vi "Destroy Events - Common GUI v3.vi"(11 "Common GUI uService in":refnum<class "Common GUI v3.lvclass">) -> (0 "error out":errorcluster, 3 "Common GUI uService out":refnum<class "Common GUI v3.lvclass">)   [LabVIEW 2026, in "TALOS.lvlib" / "Common GUI v3.lvlib" / "Common GUI v3.lvclass"]
uses:
  Common GUI v3.lvclass
  Common GUI v3.lvclass/Common GUI v3.ctl
  <vilib>/event_ctls.llb/usereventprio.ctl
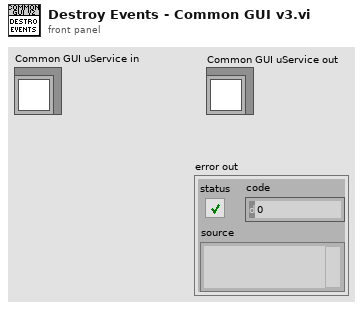
[diagram p1: front panel]
types:
  T1 = typedef "usereventprio.ctl" = enum32{"high priority", "normal priority"}
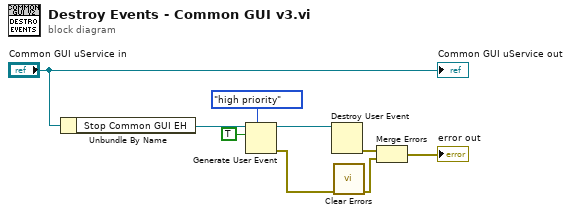
[diagram p0: block diagram]
diagram:
  n1 = Unbundle By Name("Common GUI uService in") -> ("Stop Common GUI EH"=w8:refnum<user-event>)
  n2 = Generate User Event(priority (normal)=usereventprio."high priority", user event=w8, event data cluster=TRUE ("event data")) -> (user event out=w7:refnum<user-event>, error out=w4:errorcluster)  [unwired: 1 in]
  n3 = Destroy User Event(user event=w7) -> (error out=w1:errorcluster)  [unwired: 1 in]
  n4 = call <vilib>:"Clear Errors.vi"("error in (no error)"=w4) -> ("error out"=w3:errorcluster)  [unwired: 5 in, 1 out]
  n5 = Merge Errors(w1, w3) -> (→"error out":errorcluster)
  "Common GUI uService out" <- "Common GUI uService in"
